vi "Advance past whitespace and comma.vi"(7 "JSON":string, 9 "Offset":i32, 11 "State in":T1=enum."Leading Whitespace") -> (0 "Comma Not Found":bool, 1 "Offset past match":i32, 3 "State":T1=enum."Value end")   [LabVIEW 2024, in "JSONtext.lvlib"]
uses:
  JSONtext.lvlib
  Parsing State.ctl
  Advance past Line Ending.vi
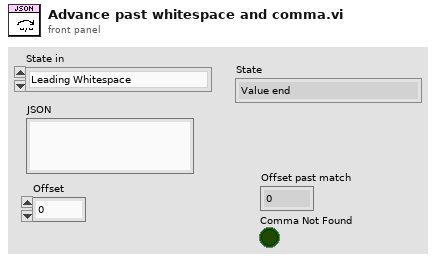
[diagram p1: front panel]
types:
  T1 = typedef "JSONtext.lvlib/Parsing State.ctl" = enum16{"Parser Error", "Object", "Array", "String", "Number/Other", "Leading Whitespace", "Object end", "Array end", "Value end"}
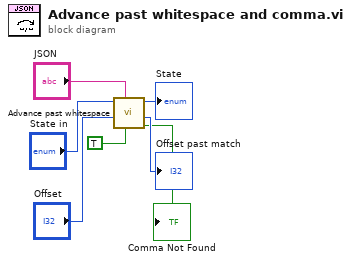
[diagram p0: block diagram]
diagram:
  n1 = call "Advance past whitespace.vi"("Past Comma"=TRUE ("Allow Comma"), "JSON"="JSON", "Offset"="Offset", "Parser State in"="State in") -> ("Comma Not Found"=→"Comma Not Found":bool, "Offset of first non-whitespace"=→"Offset past match":i32, "Parser State"=→"State":T1)  [unwired: 5 in]
